vi "EXA shm log Event State Changed LV.vi"(8 "error in (no error)":errorcluster, 11 "logevent_StateChanged_Ctl":cluster{"newState":i32, "priority":i32}) -> (0 "error out":errorcluster, 2 "function return":i32, 3 "logevent_StateChanged_Ctl out":cluster{"newState":i32, "priority":i32})   [LabVIEW 2016, in "SALLV_EXA.lvlib"]
doc: "int EXA_shm_logEvent_StateChangedLV(EXA_logevent_StateChangedLV *logevent_StateChanged_Ctl );"
uses:
  SALLV_EXA.lvlib
  SALLV_EXA.so
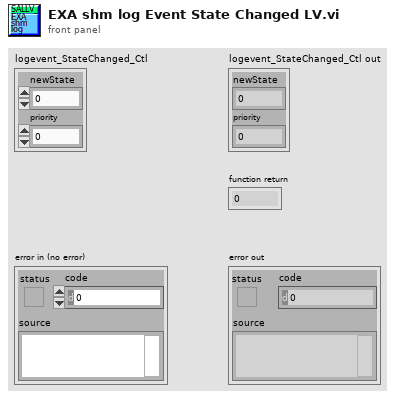
[diagram p1: front panel]
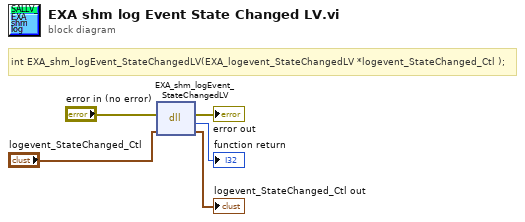
[diagram p0: block diagram]
diagram:
  # "int EXA_shm_logEvent_StateChangedLV(EXA_logevent_StateChangedLV *logevent_StateChanged_Ctl );"
  n1 = dll-call lib="home/plotz/SALLV_EXA/SALLV_EXA.*" fn="EXA_shm_logEvent_StateChangedLV"(error in="error in (no error)", "logevent_StateChanged_Ctl"="logevent_StateChanged_Ctl") -> (error out=→"error out":errorcluster, →"function return":i32, "logevent_StateChanged_Ctl"=→"logevent_StateChanged_Ctl out":cluster{"newState":i32, "priority":i32})  [unwired: 2 in, 1 out]
